vi "gen from bitfile action.vi"(8 "error in":errorcluster, 9 "user event":T1, 10 "engine configuration in":refnum<class "engine configuration.lvclass">, 11 "io configuration in":refnum<class "io configuration.lvclass">) -> (0 "error out":errorcluster, 2 "engine configuration out":refnum<class "engine configuration.lvclass">, 3 "io configuration out":refnum<class "io configuration.lvclass">)   [LabVIEW 2015, in "io editor node.lvclass"]
uses:
  io editor node.lvclass
  <vilib>/NI/Module Execution Interface/Engine Configuration/engine configuration.lvclass
  <vilib>/NI/Configuration Framework/Node/UserEventRef.ctl
  <vilib>/NI/Configuration Framework/Controls/EventCluster.ctl
  configuration/io configuration.lvclass
  configuration/io configuration.lvclass/io configuration.ctl
  <vilib>/NI/Configuration Framework/serializable configuration/NISE_CEF_serializable configuration.lvclass/NISE_CEF_serializable configuration.ctl
  <vilib>/Utility/LVClass/Get LV Class Name.vi
  <vilib>/NI/Configuration Framework/error generator/NISE_error generator.vi
  <vilib>/NI/Tag Bus Module Framework/channel/TBM channel.lvclass
  <vilib>/NI/Configuration Framework/NISE_CEF_TreeControl.lvlib
  <vilib>/NI/Configuration Framework/serializable configuration/NISE_CEF_serializable configuration.lvclass
  <vilib>/NI/Configuration Framework/Node/NISE_CEF_Node.lvclass
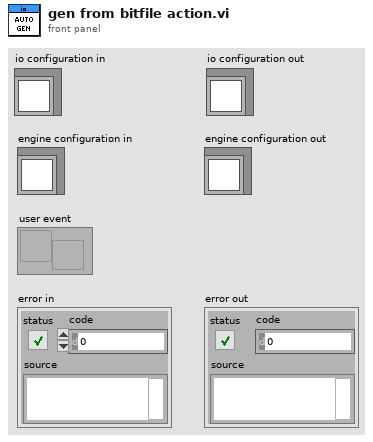
[diagram p1: front panel]
types:
  T1 = typedef "NISE_CEF_Node.lvclass/UserEventRef.ctl" = refnum<user-event>
  T2 = typedef "NISE_CEF_TreeControl.lvlib/EventCluster.ctl" = cluster{"command":string, "data":string}
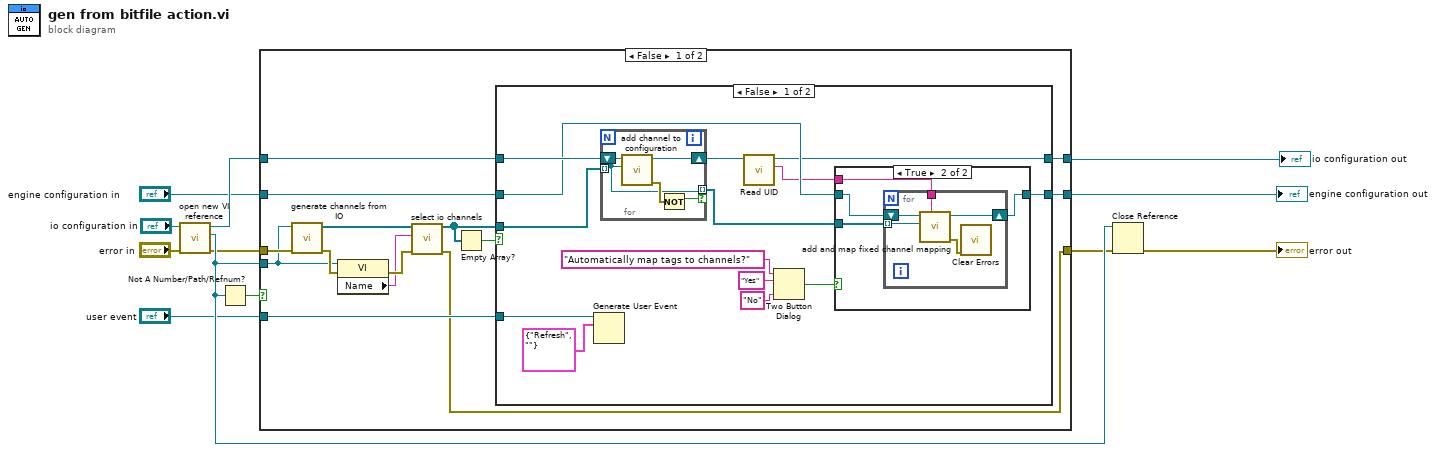
[diagram p0: block diagram]
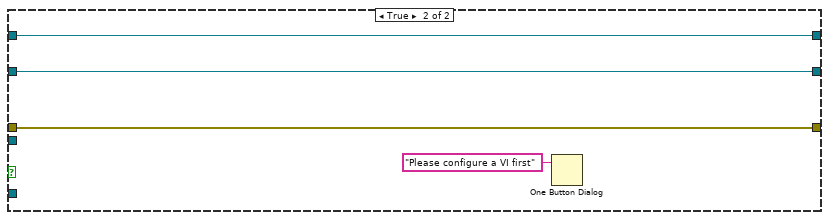
[diagram p4: hidden frame]
diagram:
  n1 = call "open new VI reference.vi"("error in"="error in", "io configuration in"="io configuration in") -> ("error out"=w8:errorcluster, "VI Refnum"=w10:refnum<vi>, "io configuration out"=w7:refnum<class "io configuration.lvclass">)  [unwired: 7 in]
  n2 = Not A Number/Path/Refnum?(number/path/refnum=w10) -> (NaN/Path/Refnum?=w3:bool)
  n3 = case shown="False" w3 {
    tunnel: w8 -> [w24 w59]
    tunnel: w7 -> [w23 w60]
    tunnel: [w21 w61] -> w12
    tunnel: "engine configuration in" -> [w22 w61]
    tunnel: [w19 w60] -> w1
    tunnel: [w13 w59] -> w5
    tunnel: w10 -> [w15 _]
    tunnel: "user event" -> [w20 _]
    frame False {
      n4 = call "generate channels from IO.vi"("error in"=w24, "VI Refnum"=w15) -> ("error out"=w26:errorcluster, "channels"=w18:refnum<class "TBM channel.lvclass">[])  [unwired: 8 in]
      n5 = property class="VI"(reference=w15, error in=w26) -> (error out=w25:errorcluster, "Name"=w14:string)  [unwired: 1 out]
      n6 = call "select io channels.vi"("error in"=w25, "API Loaded"=w14, "io channels"=w18) -> ("error out"=w13:errorcluster, "selected channels"=w16:refnum<class "TBM channel.lvclass">[])  [unwired: 7 in]
      n7 = Empty Array?(array=w16) -> (empty?=w17:bool)
      n8 = case shown="False" w17 {
        tunnel: w23 -> [w40 w57]
        tunnel: w16 -> [w39 _]
        tunnel: w22 -> [w34 w56]
        tunnel: [w33 w56] -> w21
        tunnel: w20 -> [w30 _]
        tunnel: [w28 w57] -> w19
        frame False {
          n9 = Generate User Event(user event=w30, event data cluster=T2 {"command"="Refresh", "data"=""} ("event data")) -> ()  [unwired: 2 in, 2 out]
          n10 = for {
            tunnel: w39 -> [w52] mode=indexing
            shift-right: [w54] -> w35
            shift-left: w40 -> [w55]
            tunnel: [w52] -> w32 mode=indexing if=w51
            n11 = call "add channel to configuration.vi"("channel"=w52, "io configuration in"=w55) -> ("error out"=w53:errorcluster, "io configuration out"=w54:refnum<class "io configuration.lvclass">)  [unwired: 8 in]
            n12 = Not(x=w53) -> (.not. x?=w51:bool)
          }
          n13 = call <vilib>:"Read UID.vi"("configuration in"=w35) -> ("instance id"=w27:string, "configuration out"=w28:refnum<class "io configuration.lvclass">)  [unwired: 8 in, 1 out]
          n14 = Two Button Dialog(message="Automatically map tags to channels?", 1:"No" ("F button name (\"Cancel\")"), 2:"Yes" ("T button name (\"OK\")")) -> (T button?=w36:bool)
          n15 = case shown="True" w36 {
            tunnel: w34 -> [w41 w45]
            tunnel: [w41 w44] -> w33
            tunnel: w32 -> [_ w43]
            tunnel: w27 -> [_ w42]
            frame False {
            }
            frame True {
              n16 = for {
                shift-right: [w49] -> w44
                shift-left: w45 -> [w50]
                tunnel: w43 -> [w48] mode=indexing
                tunnel: w42 -> [w46]
                n17 = call <vilib>:"add and map fixed channel mapping.vi"("module instance"=w46, "fixed channel"=w48, "engine configuration in"=w50) -> ("error out"=w47:errorcluster, "engine configuration out"=w49:refnum<class "engine configuration.lvclass">)  [unwired: 7 in]
                n18 = call <vilib>:"Clear Errors.vi"("error in (no error)"=w47) -> ()  [unwired: 5 in, 2 out]
              }
            }
          }
        }
        frame True {
        }
      }
    }
    frame True {
      n19 = One Button Dialog(message="Please configure a VI first") -> ()  [unwired: 1 in, 1 out]
    }
  }
  "engine configuration out" <- w12
  "io configuration out" <- w1
  n20 = Close Reference(reference=w10, error in (no error)=w5) -> (error out=→"error out":errorcluster)
